vi "GenerateMarvelIssuesMap.vi"(8 "error in (no error)":errorcluster, 11 "Marvel Issues map in":map{i32, T1}(c390)) -> (0 "error out":errorcluster, 3 "Marvel Issues map out":map{i32, T1}(c390))   [LabVIEW 2024]
uses:
  TypeDefs/comic--cluster.ctl
panel:
  out "current folder":string
  out "progress":i32(slide) caption="2322 of 2322" scale=0.0..2322.0
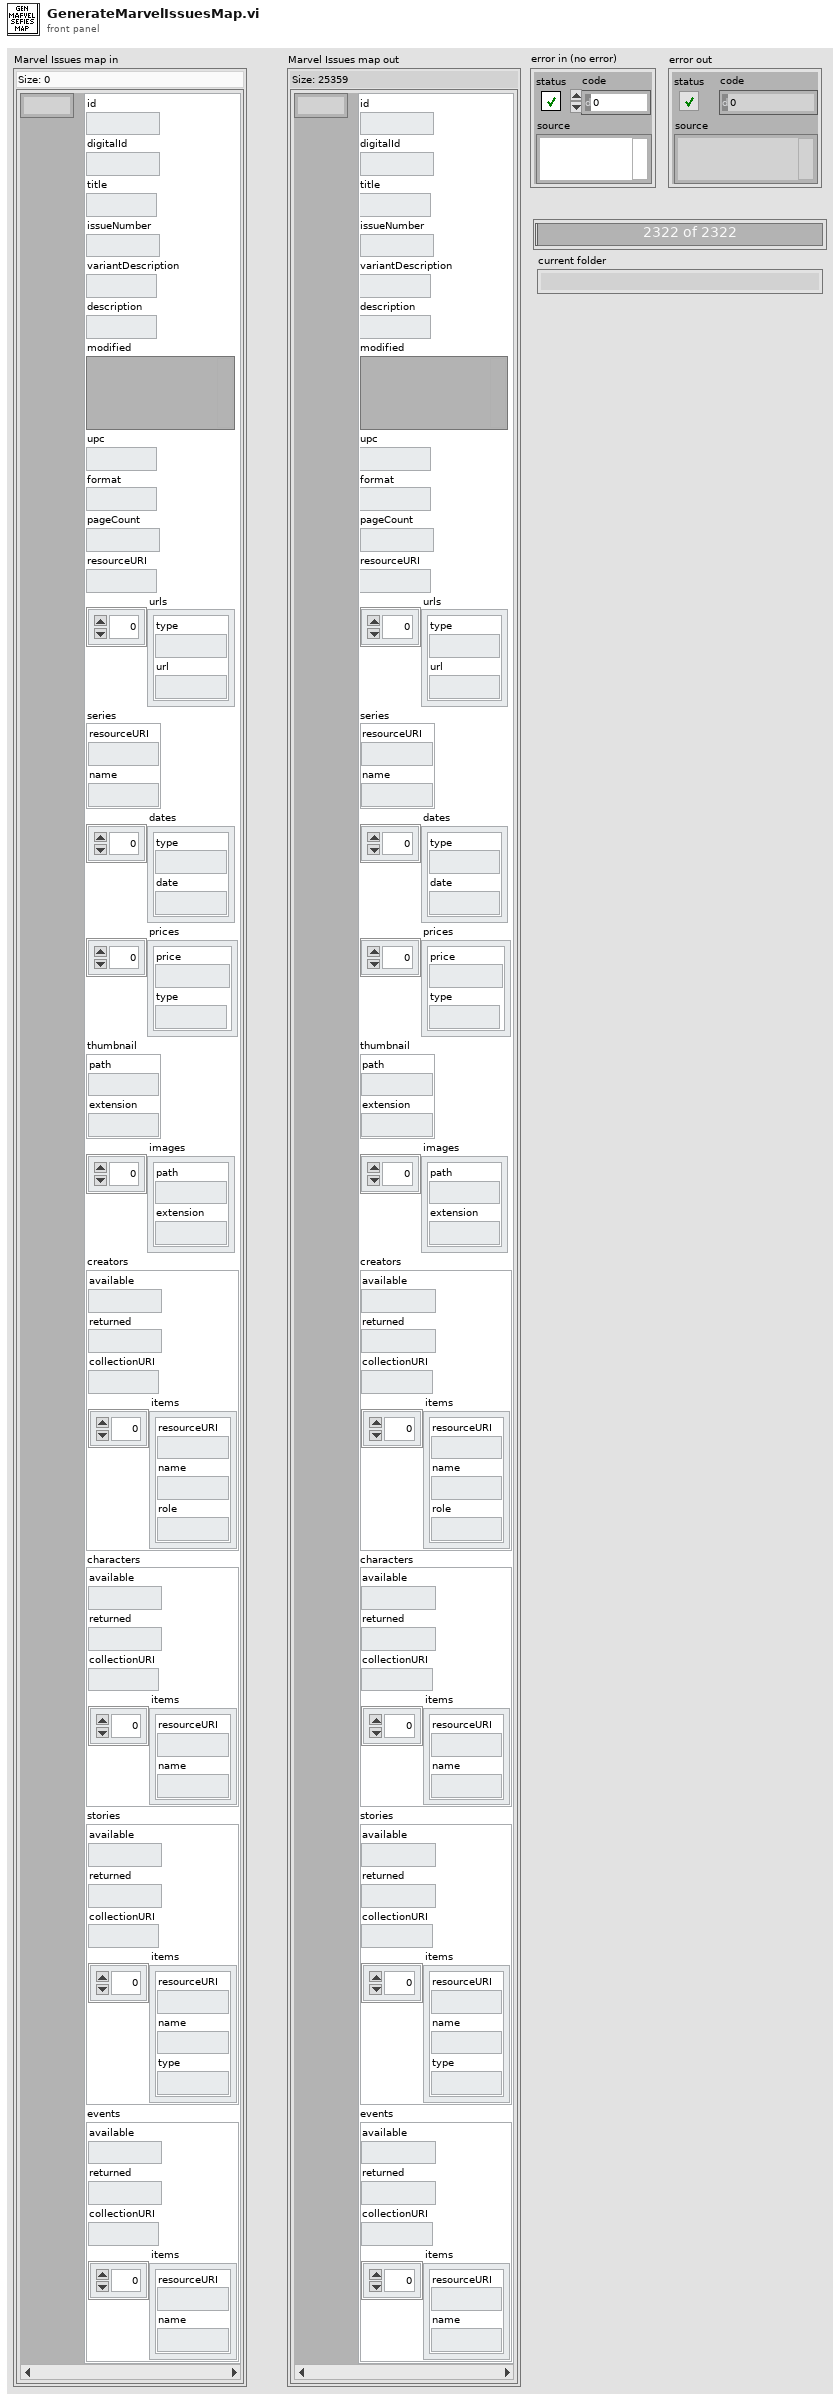
[diagram p1: front panel]
types:
  T1 = typedef "comic--cluster.ctl" = cluster{"id":i32, "digitalId":i32, "title":string, "issueNumber":i32, "variantDescription":string, "description":string, "modified":variant, "upc":string, "format":string, "pageCount":i32, "resourceURI":string, "urls":cluster{"type":string, "url":string}[], "series":cluster{"resourceURI":string, "name":string}, "dates":cluster{"type":string, "date":string}[], "prices":cluster{"price":dbl, "type":string}[], "thumbnail":cluster{"path":string, "extension":string}, "images":cluster{"path":string, "extension":string}[], "creators":cluster{"available":i32, "returned":i32, "collectionURI":string, "items":cluster{"resourceURI":string, "name":string, "role":string}[]}, "characters":cluster{"available":i32, "returned":i32, "collectionURI":string, "items":cluster{"resourceURI":string, "name":string}[]}, "stories":cluster{"available":i32, "returned":i32, "collectionURI":string, "items":cluster{"resourceURI":string, "name":string, "type":string}[]}, "events":cluster{"available":i32, "returned":i32, "collectionURI":string, "items":cluster{"resourceURI":string, "name":string}[]}}
  T2 = typedef "comics.reply--cluster.ctl" = cluster{"code":i32, "status":string, "etag":string, "data":cluster{"offset":i32, "limit":i32, "total":i32, "count":i32, "results":T1[]}}
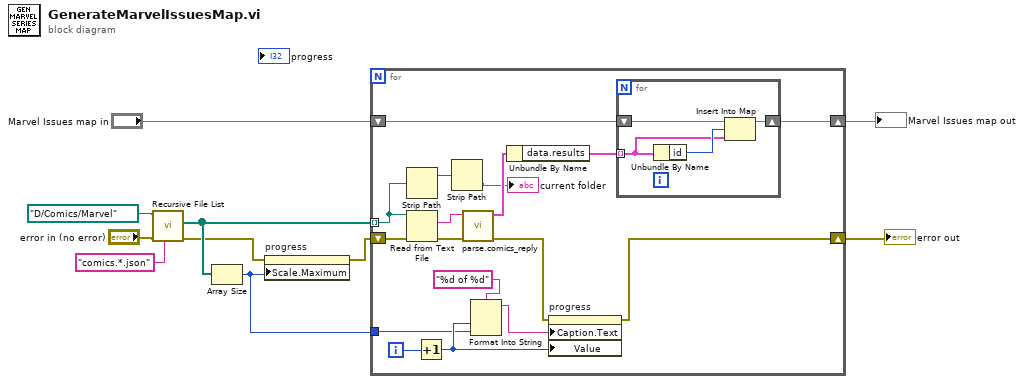
[diagram p0: block diagram]
diagram:
  n1 = call <vilib>:"Recursive File List.vi"("pattern"="comics.*.json", "error in (no error)"="error in (no error)", "Folder Path"=path "D:/Comics/Marvel") -> ("error out"=w3:errorcluster, "All Files in Dir"=w4:path[])  [unwired: 4 in, 3 out]
  n2 = Array Size(array=w4) -> (size(s)=w1:i32)
  n3 = property on="progress" class="Slide (strict)"(error in=w3, "Scale.Maximum"=w1) -> (error out=w2:errorcluster)  [unwired: 1 in, 1 out]
  n4 = for {
    tunnel: w4 -> [w13] mode=indexing
    shift-right: [w14] -> w5
    shift-left: w2 -> [w24]
    shift-right: [w26] -> w6
    shift-left: "Marvel Issues map in" -> [w27]
    tunnel: w1 -> [w17]
    i -> [w20]
    n5 = Strip Path(path=w13) -> (stripped path=w12:path)  [unwired: 1 out]
    n6 = Read from Text File(file (use dialog)=w13, error in=w24) -> (text=w23:string, error out=w25:errorcluster)  [unwired: 2 in, 2 out]
    n7 = Increment(x=w20) -> (x+1=w18:i32)
    n8 = Strip Path(path=w12) -> (name=→"current folder":string)  [unwired: 1 out]
    n9 = call "parse.comics_reply.vi"("error in"=w25, "string in"=w23) -> ("error out"=w15:errorcluster, "data"=w22:T2)  [unwired: 8 in]
    n10 = Format Into String(format string="%d of %d", w18, w17) -> (resulting string=w16:string)  [unwired: 2 in, 1 out]
    n11 = Unbundle By Name(w22) -> ("data.results"=w21:T1[])
    n12 = property on="progress" class="Slide (strict)"(error in=w15, "Caption.Text"=w16, "Value"=w18) -> (error out=w14:errorcluster)  [unwired: 1 in, 1 out]
    n13 = for {
      shift-right: [w30] -> w26
      shift-left: w27 -> [w31]
      tunnel: w21 -> [w28] mode=indexing
      n14 = Unbundle By Name(w28) -> ("id"=w29:i32)
      n15 = Insert Into Map(map in=w31, key=w29, value=w28) -> (map out=w30:map{i32, T1})  [unwired: 2 out]
    }
  }
  "Marvel Issues map out" <- w6
  "error out" <- w5
